vi "PLC.Check Enabled State.vi"(8 "error in (no error)":errorcluster, 11 "Config Folder":path=path "C:/MTE/Circle Test/Config") -> (0 "error out":errorcluster, 2 "Type":T1=enum."Dial 750", 3 "Enabled":bool)   [LabVIEW 2018]
uses:
  PLC.Type.ctl
  <vilib>/Utility/config.llb/Read Key (Boolean).vi
  <vilib>/Utility/config.llb/Read Key (String).vi
  <vilib>/Utility/config.llb/NI_LVConfig.lvlib
  <vilib>/KATE/Files/File Utils.lvlib
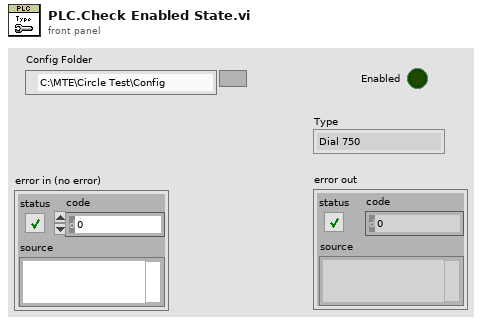
[diagram p1: front panel]
types:
  T1 = typedef "PLC.Type.ctl" = enum16{"None", "Dial 750", "Dial 800"}
  T2 = typedef "NI_LVConfig.lvlib/Config Data RefNum.ctl" = refnum<k1>
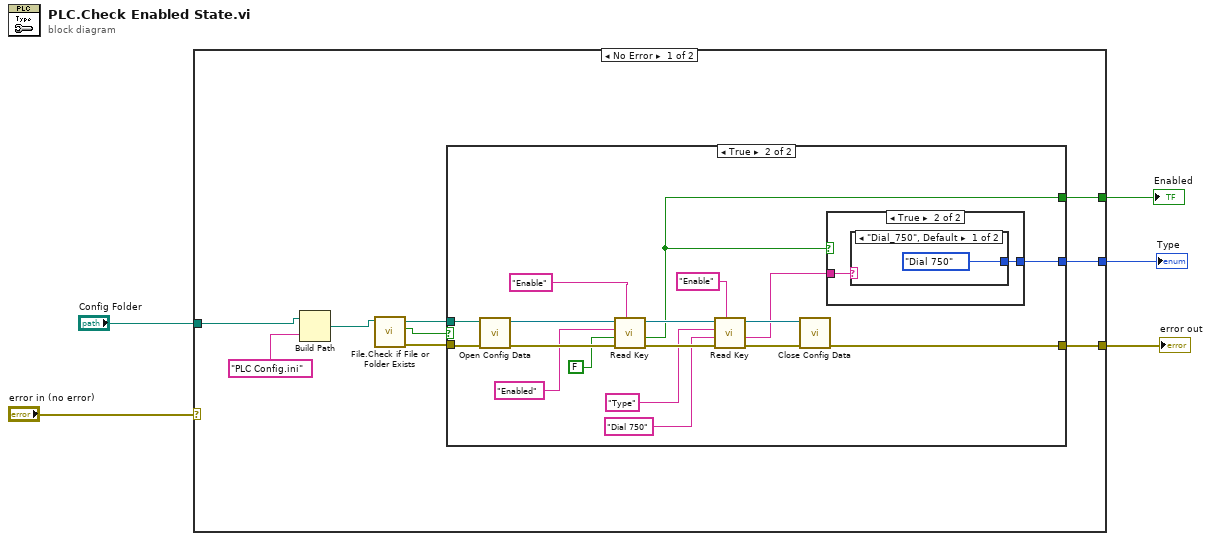
[diagram p0: block diagram]
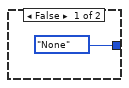
[diagram p2: hidden frame]
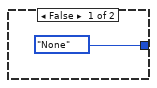
[diagram p3: hidden frame]
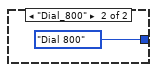
[diagram p4: hidden frame]
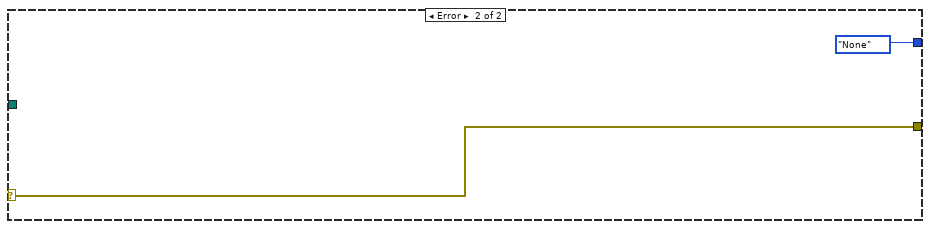
[diagram p5: hidden frame]
diagram:
  n1 = case shown="No Error" "error in (no error)" {
    selector: "error in (no error)" -> [_ w40]
    tunnel: [w14 w40] -> w4
    tunnel: "Config Folder" -> [w13 _]
    tunnel: [w11 _] -> w2
    tunnel: [w6 PLC.Type."None" ("Type")] -> w1
    frame No Error {
      n2 = Build Path(base path=w13, name or relative path="PLC Config.ini") -> (appended path=w10:path)
      n3 = call <vilib>:"File.Check if File or Folder Exists.vi"("Path"=w10) -> ("error out"=w7:errorcluster, "Exists"=w8:bool, "Dup Path"=w9:path)  [unwired: 6 in, 2 out]
      n4 = case shown="True" w8 {
        tunnel: [_ w31] -> w14
        tunnel: [_ w20] -> w11
        tunnel: w9 -> [_ w27]
        tunnel: w7 -> [_ w16]
        tunnel: [PLC.Type."None" ("Type") w21] -> w6
        frame False {
        }
        frame True {
          n5 = call <vilib>:"Open Config Data.vi"("error in (no error)"=w16, "configuration file path"=w27) -> ("error out"=w33:errorcluster, "refnum"=w32:T2)  [unwired: 7 in, 1 out]
          n6 = call-poly <vilib>:"Read Key.vi"("section"="Enable", "error in (no error)"=w33, "default value"=FALSE, "key"="Enabled", "refnum"=w32) -> ("error out"=w25:errorcluster, "value"=w20:bool, "refnum out"=w26:T2)  [unwired: 3 in, 1 out]
          n7 = call-poly <vilib>:"Read Key.vi"("section"="Enable", "error in (no error)"=w25, "default value"="Dial 750", "key"="Type", "refnum"=w26) -> ("error out"=w24:errorcluster, "value"=w19:string, "refnum out"=w23:T2)  [unwired: 3 in, 1 out]
          n8 = call <vilib>:"Close Config Data.vi"("error in (no error)"=w24, "refnum"=w23) -> ("error out"=w31:errorcluster)  [unwired: 8 in, 1 out]
          n9 = case shown="True" w20 {
            tunnel: [PLC.Type."None" ("Type") w36] -> w21
            tunnel: w19 -> [_ w35]
            frame False {
            }
            frame True {
              n10 = case shown="\"Dial_750\", Default" w35 {
                tunnel: [PLC.Type."Dial 750" ("Type") PLC.Type."Dial 800" ("Type")] -> w36
                frame "Dial_750", Default {
                }
                frame "Dial_800" {
                }
              }
            }
          }
        }
      }
    }
    frame Error {
    }
  }
  "error out" <- w4
  "Enabled" <- w2
  "Type" <- w1
